vi "Get or Add WorkbookStylesPart.vi"(8 "error in":errorcluster, 11 "SpreadsheetDoc in":refnum<k24>) -> (0 "error out":errorcluster, 2 "WorkbookStylesPart":refnum<k24>, 3 "SpreadsheetDoc out":refnum<k24>)   [LabVIEW 2021, in "Open Xml.lvlib"]
uses:
  Open Xml.lvlib
  D:/git/Open-Xml-LabVIEW/dll/DocumentFormat.OpenXml.dll
  dll/DocumentFormat.OpenXml.dll
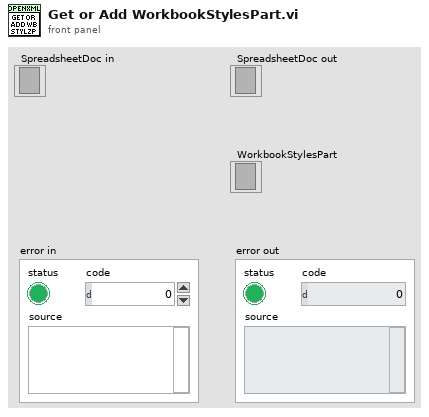
[diagram p1: front panel]
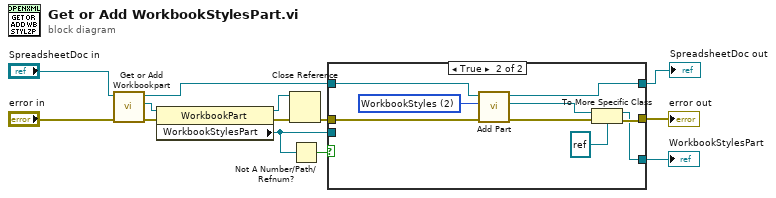
[diagram p0: block diagram]
diagram:
  n1 = call "Get or Add Workbookpart.vi"("error in"="error in", "SpreadsheetDocument"="SpreadsheetDoc in") -> ("error out"=w13:errorcluster, "WorkbookPart"=w11:refnum<k24>, "SpreadsheetDocument out"=w4:refnum<k24>)  [unwired: 7 in]
  n2 = property class="WorkbookPart"(reference=w11, error in=w13) -> (reference out=w1:refnum<k24>, error out=w9:errorcluster, "WorkbookStylesPart"=w5:refnum<k24>)
  n3 = Close Reference(reference=w1, error in (no error)=w9) -> (error out=w2:errorcluster)
  n4 = Not A Number/Path/Refnum?(number/path/refnum=w5) -> (NaN/Path/Refnum?=w7:bool)
  n5 = case shown="True" w7 {
    tunnel: w2 -> [w16 w21]
    tunnel: [w16 w25] -> w8
    tunnel: [w15 w22] -> w6
    tunnel: w5 -> [w15 _]
    tunnel: w4 -> [w14 w20]
    tunnel: [w14 w19] -> w3
    frame False {
    }
    frame True {
      w17 = 2 items=["SharedString", "Worksheet", "WorkbookStyles"] ("partType")
      n6 = call "Add Part.vi"("error in"=w21, "PartType"=w17, "SpreadsheetDocument in"=w20) -> ("error out"=w18:errorcluster, "OpenXmlPart"=w23:refnum<k24>, "SpreadsheetDocument out"=w19:refnum<k24>)  [unwired: 6 in]
      n7 = To More Specific Class(target class=refnum<k24> refnum ("WorkbookStylesPart 2"), reference=w23, error in=w18) -> (specific class reference=w22:refnum<k24>, error out=w25:errorcluster)
    }
  }
  "WorkbookStylesPart" <- w6
  "error out" <- w8
  "SpreadsheetDoc out" <- w3
